vi "Test Force Displacement.vi"(8 "error in (no error)":errorcluster, 10 "Number of Steps Commanded":i32, 11 "Model in":refnum<class "Model.lvclass">) -> (0 "error out":errorcluster, 2 "Is Force Outside of Range?":bool, 3 "Model out":refnum<class "Model.lvclass">)   [LabVIEW 2016, in "Model.lvclass"]
uses:
  Model.lvclass
  Model.lvclass/Model.ctl
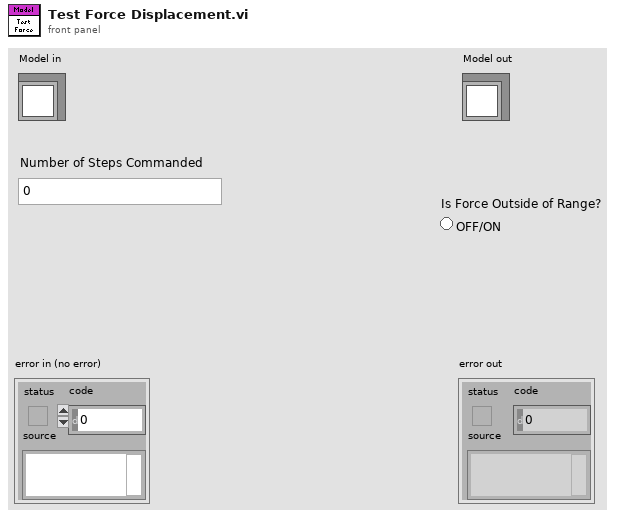
[diagram p1: front panel]
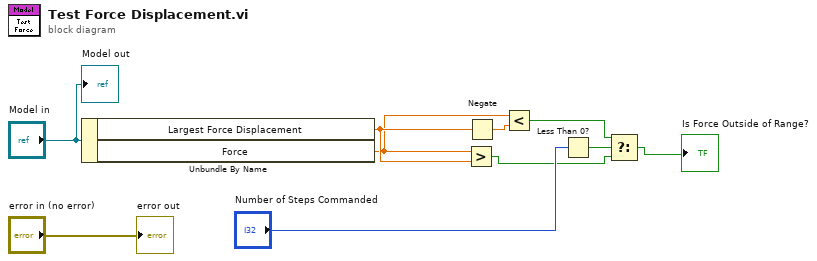
[diagram p0: block diagram]
diagram:
  n1 = Unbundle By Name("Model in") -> ("Largest Force Displacement"=w8:dbl, "Force"=w7:dbl)
  n2 = Greater?(x=w7, y=w8) -> (0:w2:bool)
  n3 = Negate(x=w8) -> (-x=w9:dbl)
  n4 = Less?(x=w7, y=w9) -> (x < y?=w3:bool)
  n5 = Less Than 0?(x="Number of Steps Commanded") -> (x < 0?=w4:bool)
  n6 = Select(t=w3, s=w4, f=w2) -> (s? t:f=→"Is Force Outside of Range?":bool)
  "error out" <- "error in (no error)"
  "Model out" <- "Model in"
